vi "initial tests.vi"() -> ()   [LabVIEW 2020]
uses:
  client/client.lvlib
panel:
  out "Array":string[](array[string])
  out "function return 2":i32
  out "function return":i32
  out "buf out":string
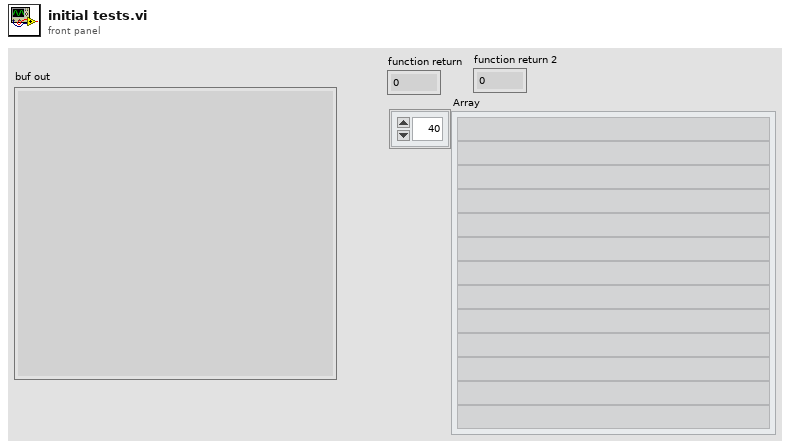
[diagram p1: front panel]
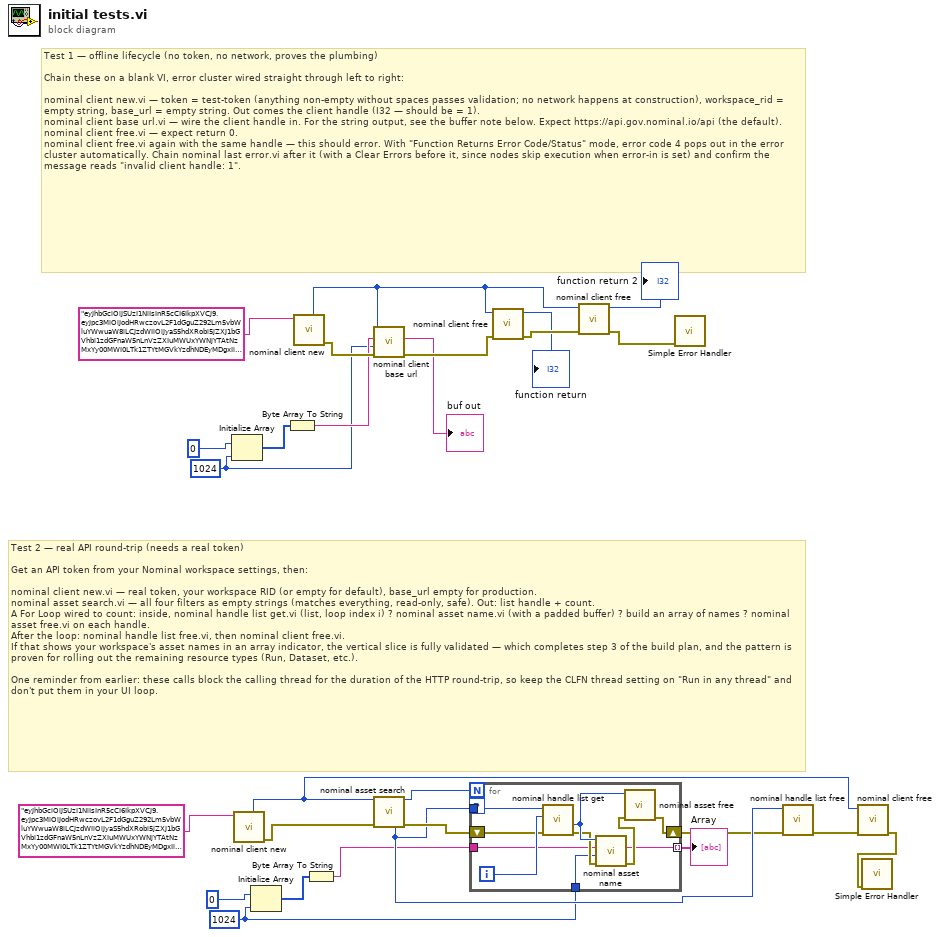
[diagram p0: block diagram]
diagram:
  w2 = 1024
  w16 = 1024
  # "Test 2 — real API round-trip (needs a real token)\n\nGet an API token from your Nominal workspace settings, then:\n\nnominal client new.vi — real token, your workspace RID (or empty for default), base_url empty for production.\nnominal asset search.vi — all four filters as empty strings (matches everything, read-only, safe). Out: list handle + count.\nA For Loop wired to count: inside, nominal handle list get.vi (list, loop index i) ? nominal asset name.vi (with a padded buffer) ? build an array of names ? nominal asset free.vi on each handle.\nAfter the loop: nominal handle list free.vi, then nominal client free.vi.\nIf that shows your workspace's asset names in an array indicator, the vertical slice is fully validated — which completes step 3 of the build plan, and the pattern is proven for rolling out the remaining resource types (Run, Dataset, etc.).\n\nOne reminder from earlier: these calls block the calling thread for the duration of the HTTP round-trip, so keep the CLFN thread setting on \"Run in any thread\" and don't put them in your UI loop."
  # "Test 1 — offline lifecycle (no token, no network, proves the plumbing)\n\nChain these on a blank VI, error cluster wired straight through left to right:\n\nnominal client new.vi — token = test-token (anything non-empty without spaces passes validation; no network happens at construction), workspace_rid = empty string, base_url = empty string. Out comes the client handle (I32 — should be = 1).\nnominal client base url.vi — wire the client handle in. For the string output, see the buffer note below. Expect https://api.gov.nominal.io/api (the default).\nnominal client free.vi — expect return 0.\nnominal client free.vi again with the same handle — this should error. With \"Function Returns Error Code/Status\" mode, error code 4 pops out in the error cluster automatically. Chain nominal last error.vi after it (with a Clear Errors before it, since nodes skip execution when error-in is set) and confirm the message reads \"invalid client handle: 1\"."
  n1 = Initialize Array(u8 0, w16) -> (w15:u8[])
  n2 = call "nominal client new.vi"("token"="eyJhbGciOiJSUzI1NiIsInR5cCI6IkpXVCJ9.eyJpc3MiOiJodHRwczovL2F1dGguZ292Lm5vbWluYWwuaW8iLCJzdWIiOiJyaS5hdXRobi5jZXJ1bGVhbi1zdGFnaW5nLnVzZXIuMWUxYWNjYTAtNzMxYy00MWI0LTk1ZTYtMGVkYzdhNDEyMDgxIiwibm9taW5hbCI6eyJ1c2VyX3V1aWQiOiIxZTFhY2NhMC03MzFjLTQxYjQtOTVlNi0wZWRjN2E0MTIwODEiLCJvcmdhbml6YXRpb25fdXVpZCI6IjdkODAyZDRlLTdmMWMtNDViOS1iYTA1LWY3ZjYzMjM1MDRkNiIsInNjb3BlIjpbIlRydWVTY29wZSIsIklOU1RBTkNFIl19LCJleHAiOjE3ODYyMTg5MzEsImF1ZCI6Imh0dHBzOi8vYXBpLmdvdi5ub21pbmFsLmlvIn0.b1R-OTsEoXRBlxRscJn3Ag9EOYiyqHQjGKv9pTBUhInJclWOAX28gvJz6cmUxBR8ljVp-rSapiHV0CRGFIIfuFzaXlOXcd2GntvPqV_t5DapkDu1kJ_iQYTfrrD3NJUE9koxTrQHBzkmhIsGH21lGLaq9QIc0FltD4EptmGRrGEB99Q3zXbogZFfbscLU9-j1OiblutRKnsmUv2SOjkWYxjMdhkNGo9NB-b5njzqYCn1Mr8s0p7PsnblL-QoPUUUEMQgUzGOgtDotBPYajRze-E-Tir02zbfpKdple5wSNXtveaNR1N9fXXWzJleehOcnRYrykIDFXTw7A8GnLvJvQ") -> ("error out"=w11:errorcluster, "out_client out"=w7:i32)  [unwired: 8 in, 1 out]
  n3 = Initialize Array(u8 0, w2) -> (w4:u8[])
  n4 = Byte Array To String(unsigned byte array=w15) -> (string=w18:string)
  n5 = call "nominal client new.vi"("token"="eyJhbGciOiJSUzI1NiIsInR5cCI6IkpXVCJ9.eyJpc3MiOiJodHRwczovL2F1dGguZ292Lm5vbWluYWwuaW8iLCJzdWIiOiJyaS5hdXRobi5jZXJ1bGVhbi1zdGFnaW5nLnVzZXIuMWUxYWNjYTAtNzMxYy00MWI0LTk1ZTYtMGVkYzdhNDEyMDgxIiwibm9taW5hbCI6eyJ1c2VyX3V1aWQiOiIxZTFhY2NhMC03MzFjLTQxYjQtOTVlNi0wZWRjN2E0MTIwODEiLCJvcmdhbml6YXRpb25fdXVpZCI6IjdkODAyZDRlLTdmMWMtNDViOS1iYTA1LWY3ZjYzMjM1MDRkNiIsInNjb3BlIjpbIlRydWVTY29wZSIsIklOU1RBTkNFIl19LCJleHAiOjE3ODYyMTg5MzEsImF1ZCI6Imh0dHBzOi8vYXBpLmdvdi5ub21pbmFsLmlvIn0.b1R-OTsEoXRBlxRscJn3Ag9EOYiyqHQjGKv9pTBUhInJclWOAX28gvJz6cmUxBR8ljVp-rSapiHV0CRGFIIfuFzaXlOXcd2GntvPqV_t5DapkDu1kJ_iQYTfrrD3NJUE9koxTrQHBzkmhIsGH21lGLaq9QIc0FltD4EptmGRrGEB99Q3zXbogZFfbscLU9-j1OiblutRKnsmUv2SOjkWYxjMdhkNGo9NB-b5njzqYCn1Mr8s0p7PsnblL-QoPUUUEMQgUzGOgtDotBPYajRze-E-Tir02zbfpKdple5wSNXtveaNR1N9fXXWzJleehOcnRYrykIDFXTw7A8GnLvJvQ") -> ("error out"=w26:errorcluster, "out_client out"=w27:i32)  [unwired: 8 in, 1 out]
  n6 = Byte Array To String(unsigned byte array=w4) -> (string=w3:string)
  n7 = call "nominal client base url.vi"("error in (no error)"=w26, "cap"=w16, "buf"=w18, "client"=w27) -> ("error out"=w25:errorcluster, "buf out"=→"buf out":string)  [unwired: 4 in, 2 out]
  n8 = call "nominal asset search.vi"("client"=w7, "error in (no error)"=w11) -> ("out_count out"=w13:u32, "out_list out"=w10:i32, "error out"=w12:errorcluster)  [unwired: 10 in, 1 out]
  n9 = for {
    N: w13 -> [_]
    tunnel: w10 -> [w37]
    shift-right: [w31] -> w9
    shift-left: w12 -> [w32]
    tunnel: w3 -> [w30]
    tunnel: w2 -> [w29]
    tunnel: [w28] -> w1 mode=indexing
    workers-P: _ -> [_]
    i -> [w35]
    n10 = call "nominal handle list get.vi"("error in (no error)"=w32, "index"=w35, "list"=w37) -> ("error out"=w33:errorcluster, "out_handle out"=w36:i32)  [unwired: 6 in, 1 out]
    n11 = call "nominal asset name.vi"("error in (no error)"=w33, "cap"=w29, "buf"=w30, "asset"=w36) -> ("error out"=w34:errorcluster, "buf out"=w28:string)  [unwired: 4 in, 2 out]
    n12 = call "nominal asset free.vi"("error in (no error)"=w34, "asset"=w36) -> ("error out"=w31:errorcluster)  [unwired: 8 in, 1 out]
  }
  "Array" <- w1
  n13 = call "nominal client free.vi"("error in (no error)"=w25, "client"=w27) -> ("error out"=w24:errorcluster, "function return"=→"function return":i32)  [unwired: 8 in]
  n14 = call "nominal client free.vi"("error in (no error)"=w24, "client"=w27) -> ("error out"=w21:errorcluster, "function return"=→"function return 2":i32)  [unwired: 8 in]
  n15 = call <vilib>:"Simple Error Handler.vi"("error in (no error)"=w21) -> ()  [unwired: 4 in, 5 out]
  n16 = call "nominal handle list free.vi"("error in (no error)"=w9, "list"=w10) -> ("error out"=w8:errorcluster)  [unwired: 8 in, 1 out]
  n17 = call "nominal client free.vi"("error in (no error)"=w8, "client"=w7) -> ("error out"=w6:errorcluster)  [unwired: 8 in, 1 out]
  n18 = call <vilib>:"Simple Error Handler.vi"("error in (no error)"=w6) -> ()  [unwired: 4 in, 5 out]
